vi "周期设置_氨氮.vi"() -> ()   [LabVIEW 2016, in "斯坦道氨氮.lvlib"]
uses:
  <vilib>/Utility/miscctls.llb/LVPointTypeDef.ctl
  <vilib>/Utility/config.llb/NI_LVConfig.lvlib
panel:
  in  "运行周期":T1={"运行模式"=enum."维护模式", "质控频次"=enum."关闭", "空白核查时间"=2, "跨度核查时间"=6, "24H周期设置"=[]} {"跨度核查时间" items=["00H", "01H", "02H", "03H", "04H", "05H", "06H", "07H", "08H", "09H", "10H", "11H", "12H", "13H", "14H", "15H", "16H", "17H", "18H", "19H", "20H", "21H", "22H", "23H", "关闭"]; "空白核查时间" items=["00H", "01H", "02H", "03H", "04H", "05H", "06H", "07H", "08H", "09H", "10H", "11H", "12H", "13H", "14H", "15H", "16H", "17H", "18H", "19H", "20H", "21H", "22H", "23H", "关闭"]}
  # "运行模式："
  # "质控频次："
  # "空白核查时间："
  # "跨度核查时间："
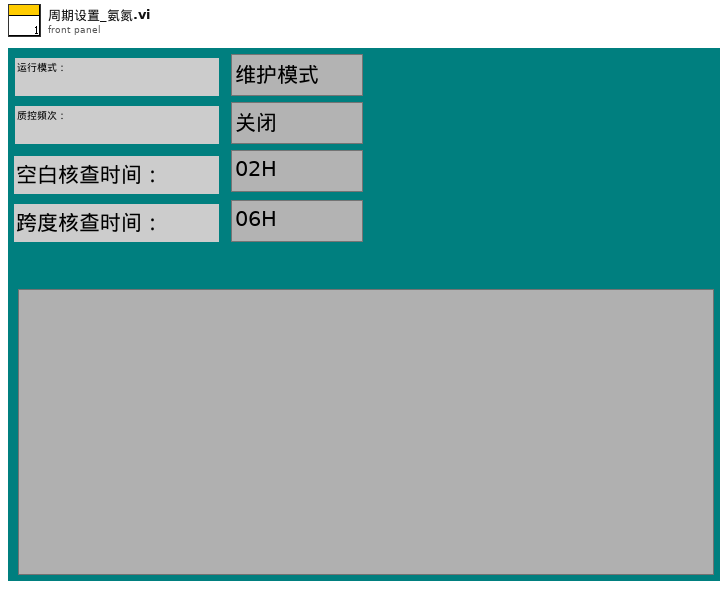
[diagram p1: front panel]
types:
  T1 = cluster{"运行模式":enum16{"维护模式", "常规模式", "应急模式", "质控模式"}, "质控频次":enum16{"关闭", "每天", "星期一", "星期二", "星期三", "星期四", "星期五", "星期六", "星期日"}, "空白核查时间":u16, "跨度核查时间":u16, "24H周期设置":bool[]}
  T2 = typedef "LVPointTypeDef.ctl" = cluster{"Horizontal":i16, "Vertical":i16}
  T3 = cluster{"站号":u16, "量程切换":enum32{"H", "L", "AUTO"}, "控制命令":enum16{"启动测量", "标样核查", "零点核查", "跨度核查", "空白测试", "平行样测试", "加标回收", "空白校准", "标样校准", "初始化（清洗）", "停止测试", "仪器重启", "校时", "模式设置", "测量间隔设置"}, "模式设置":enum16{"待机", "连续模式", "周期模式", "定点模式", "受控模式", "手动模式"}, "测量间隔":u16}
  T4 = enum16{"启动测量", "标样核查", "零点核查", "跨度核查", "空白测试", "平行样测试", "加标回收", "空白校准", "标样校准", "初始化（清洗）", "停止测试", "仪器重启", "校时", "模式设置", "测量间隔设置"}
  T5 = enum16{"关闭", "每天", "星期一", "星期二", "星期三", "星期四", "星期五", "星期六", "星期日"}
  T6 = typedef "LVDateTimeRec.ctl" = cluster{"秒数的小数部分":dbl, "秒":i32, "分":i32, "时":i32, "日":i32, "月":i32, "年":i32, "天数（周）":i32, "天数（年）":i32, "DST":i32}
  T7 = enum32{"Bad", "Idle", "Run top level", "Running"}
  T8 = cluster{"水样测试量程模式":enum16{"H", "L", "AUTO"}, "空白核查量程模式":enum16{"H", "L", "AUTO"}, "跨度核查量程模式":enum16{"H", "L", "AUTO"}}
  T9 = typedef "NI_LVConfig.lvlib/Config Data RefNum.ctl" = refnum<k1>
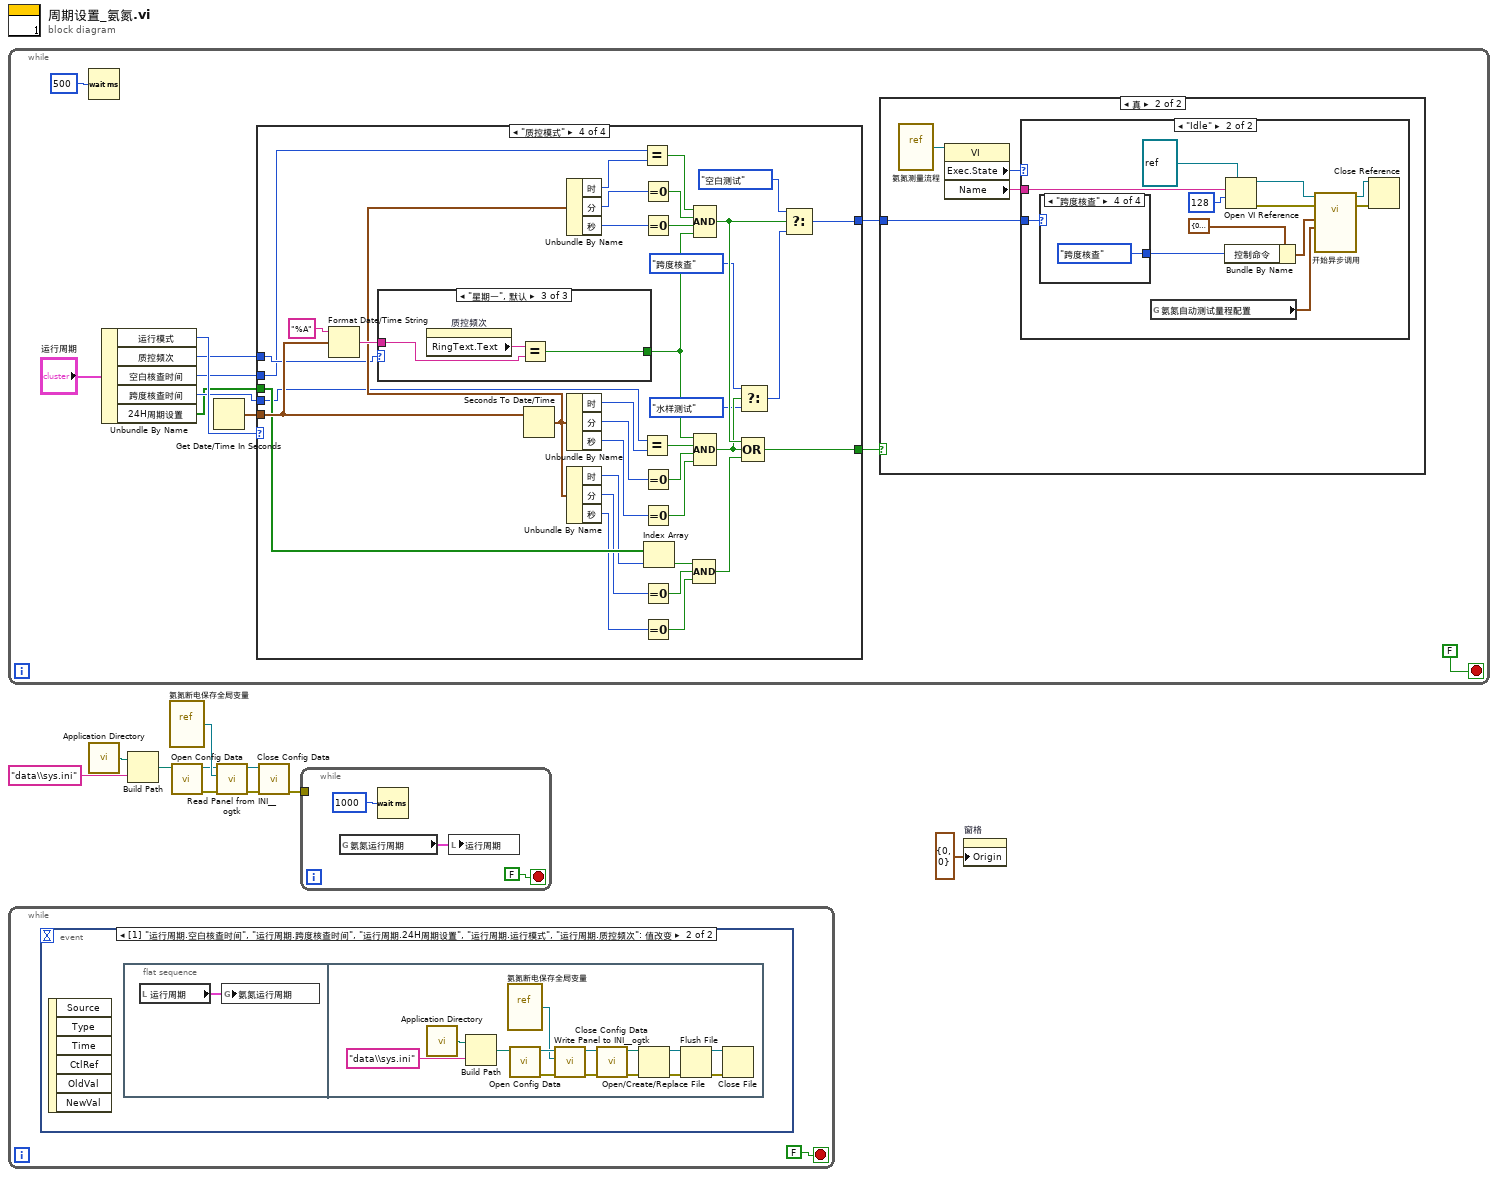
[diagram p0: block diagram]
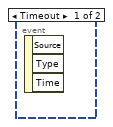
[diagram p2: hidden frame]
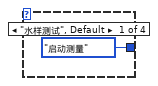
[diagram p5: hidden frame]
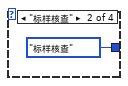
[diagram p6: hidden frame]
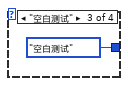
[diagram p7: hidden frame]
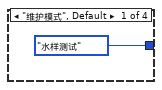
[diagram p8: hidden frame]
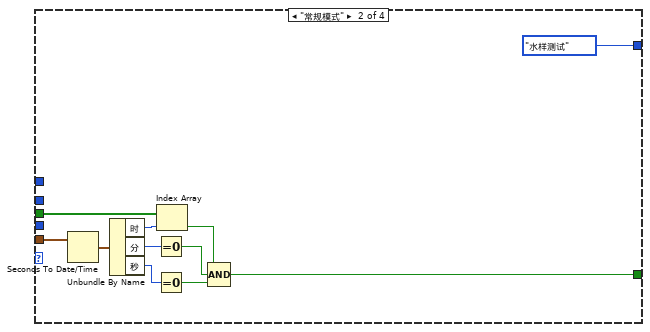
[diagram p9: hidden frame]
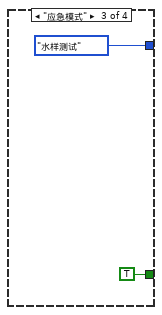
[diagram p10: hidden frame]
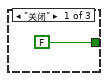
[diagram p11: hidden frame]
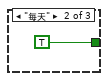
[diagram p12: hidden frame]
diagram:
  n1 = while {
    stop <- FALSE stop-if-true
    n2 = Wait (ms)(milliseconds to wait=u32 500 ("等待时间（毫秒）")) -> ()  [unwired: 1 out]
    n3 = Unbundle By Name("运行周期") -> ("运行模式"=w15:enum16{"维护模式", "常规模式", "应急模式", "质控模式"}, "质控频次"=w14:T5, "空白核查时间"=w13:u16, "跨度核查时间"=w12:u16, "24H周期设置"=w11:bool[])
    n4 = Get Date/Time In Seconds() -> (seconds since 1Jan1904=w21:timestamp)
    n5 = case shown="\"质控模式\"" w15 {
      tunnel: w21 -> [_ w52 _ w91]
      tunnel: w11 -> [_ w49 _ w88]
      tunnel: [_ w43 TRUE w68] -> w18
      tunnel: [enum16{"水样测试", "标样核查", "空白测试", "跨度核查"}."水样测试" ("仪器测试类型") enum16{"水样测试", "标样核查", "空白测试", "跨度核查"}."水样测试" ("仪器测试类型") enum16{"水样测试", "标样核查", "空白测试", "跨度核查"}."水样测试" ("仪器测试类型") w61] -> w17
      tunnel: w14 -> [_ _ _ w58]
      tunnel: w13 -> [_ _ _ w57]
      tunnel: w12 -> [_ _ _ w56]
      frame "维护模式", Default {
      }
      frame "常规模式" {
        n6 = Seconds To Date/Time(time stamp (now)=w52) -> (date time rec=w51:T6)  [unwired: 1 in]
        n7 = Unbundle By Name(w51) -> ("时"=w50:i32, "分"=w48:i32, "秒"=w47:i32)
        n8 = Equal To 0?(x=w48) -> (x = 0?=w45:bool)
        n9 = Equal To 0?(x=w47) -> (x = 0?=w44:bool)
        n10 = Index Array(array=w49, index=w50) -> (element=w46:bool)
        n11 = Compound Arithmetic op=AND ("复合运算")(w46, w45, w44) -> (w43:bool)
      }
      frame "应急模式" {
      }
      frame "质控模式" {
        n12 = Format Date/Time String(time format string (%c)="%A" ("时间格式字符串(%c)"), seconds (now)=w91) -> (date/time string=w89:string)  [unwired: 1 in]
        n13 = case shown="\"星期一\", 默认" w58 {
          tunnel: w89 -> [_ _ w95]
          tunnel: [FALSE TRUE w94] -> w59
          frame "关闭" {
          }
          frame "每天" {
          }
          frame "星期一", Default {
            n14 = property on="质控频次" class="Enum (严格)"() -> ("RingText.Text"=w96:string)  [unwired: 2 in, 2 out]
            n15 = Equal?(x=w96, y=w95) -> (x = y?=w94:bool)
          }
        }
        n16 = Seconds To Date/Time(time stamp (now)=w91) -> (date time rec=w72:T6)  [unwired: 1 in]
        n17 = Unbundle By Name(w72) -> ("时"=w81:i32, "分"=w80:i32, "秒"=w79:i32)
        n18 = Unbundle By Name(w72) -> ("时"=w73:i32, "分"=w74:i32, "秒"=w75:i32)
        n19 = Unbundle By Name(w72) -> ("时"=w87:i32, "分"=w85:i32, "秒"=w83:i32)
        n20 = Equal?(x=w57, y=w81) -> (x = y?=w78:bool)
        n21 = Equal?(x=w56, y=w73) -> (x = y?=w71:bool)
        n22 = Equal To 0?(x=w80) -> (x = 0?=w77:bool)
        n23 = Equal To 0?(x=w79) -> (x = 0?=w76:bool)
        n24 = Equal To 0?(x=w74) -> (x = 0?=w70:bool)
        n25 = Equal To 0?(x=w75) -> (x = 0?=w69:bool)
        n26 = Equal To 0?(x=w85) -> (x = 0?=w84:bool)
        n27 = Equal To 0?(x=w83) -> (x = 0?=w82:bool)
        n28 = Index Array(array=w88, index=w87) -> (element=w86:bool)
        n29 = Compound Arithmetic op=AND ("复合运算")(w86, w84, w82) -> (w60:bool)
        n30 = Compound Arithmetic op=AND ("复合运算")(w78, w77, w76, w59) -> (w67:bool)
        n31 = Compound Arithmetic op=AND ("复合运算")(w59, w71, w70, w69) -> (w65:bool)
        n32 = Select(t=enum16{"水样测试", "标样核查", "空白测试", "跨度核查"}."跨度核查" ("仪器测试类型"), s=w65, f=enum16{"水样测试", "标样核查", "空白测试", "跨度核查"}."水样测试" ("仪器测试类型")) -> (s? t:f=w63:enum16{"水样测试", "标样核查", "空白测试", "跨度核查"})
        n33 = Compound Arithmetic op=OR ("复合运算")(w67, w65, w60) -> (w68:bool)
        n34 = Select(t=enum16{"水样测试", "标样核查", "空白测试", "跨度核查"}."空白测试" ("仪器测试类型"), s=w67, f=w63) -> (s? t:f=w61:enum16{"水样测试", "标样核查", "空白测试", "跨度核查"})
      }
    }
    n35 = case shown="真" w18 {
      tunnel: w17 -> [_ w22]
      frame False {
      }
      frame True {
        n36 = vi-ref "氨氮测量流程.vi"() -> (w23:refnum<vi>)
        n37 = property class="VI"(reference=w23) -> ("Exec.State"=w25:T7, "Name"=w24:string)  [unwired: 1 in, 2 out]
        n38 = case shown="\"Idle\"" w25 {
          tunnel: w24 -> [_ w32]
          tunnel: w22 -> [_ w26]
          frame "Bad", Default {
          }
          frame "Idle" {
            n39 = case shown="\"跨度核查\"" w26 {
              tunnel: [T4."启动测量" ("控制命令") T4."标样核查" ("控制命令") T4."空白测试" ("控制命令") T4."跨度核查" ("控制命令")] -> w28
              frame "水样测试", Default {
              }
              frame "标样核查" {
              }
              frame "空白测试" {
              }
              frame "跨度核查" {
              }
            }
            n40 = global read "氨氮断电保存全局变量.vi" "氨氮自动测试量程配置"() -> (w27:T8)
            n41 = Bundle By Name(cluster=T3 {"站号"=0, "量程切换"=enum."H", "控制命令"=enum."启动测量", "模式设置"=enum."待机", "测量间隔"=0} ("参数"), "控制命令"=w28) -> (w29:T3)
            n42 = Open VI Reference(type specifier VI Refnum (for type only)=refnum<vi> refnum, vi path=w32, options=128 ("选项")) -> (vi reference=w33:refnum<vi>, error out=w34:errorcluster)  [unwired: 3 in]
            n43 = call-by-ref "开始异步调用"(reference=w33, error in=w34, "量程模式"=w27, "参数"=w29) -> (reference out=w35:refnum<vi>, error out=w36:errorcluster)  [unwired: 10 in]
            n44 = Close Reference(reference=w35, error in (no error)=w36) -> ()  [unwired: 1 out]
          }
        }
      }
    }
  }
  n45 = while {
    stop <- FALSE stop-if-true
    n46 = event shown="[1] \"运行周期.空白核查时间\", \"运行周期.跨度核查时间\", \"运行周期.24H周期设置\", \"运行周期.运行模式\", \"运行周期.质控频次\": 值改变" {
      selector: _ -> [_ _]
      dyn-events: _ -> [_ _]
      timeout: _ -> [_ _]
      event Timeout {
        n47 = event-data() -> ()  [unwired: 1 in, 3 out]
      }
      event "运行周期.空白核查时间", "运行周期.跨度核查时间", "运行周期.24H周期设置", "运行周期.运行模式", "运行周期.质控频次": Value Change {
        n48 = event-data() -> ()  [unwired: 1 in, 6 out]
        n49 = flat-sequence {
          frame #0 {
            n50 = local read "运行周期"() -> (w98:T1)
            n51 = global write "氨氮断电保存全局变量.vi" "氨氮运行周期"(w98) -> ()
          }
          frame #1 {
            n52 = call <vilib>:"Application Directory.vi"() -> ("Application Directory"=w112:path)
            n53 = Build Path(base path=w112, name or relative path="data\\sys.ini" ("名称或相对路径")) -> (appended path=w110:path)
            n54 = vi-ref "氨氮断电保存全局变量.vi"() -> (w108:refnum<vi>)
            n55 = call <vilib>:"Open Config Data.vi"("configuration file path"=w110) -> ("error out"=w106:errorcluster, "refnum"=w109:T9)  [unwired: 8 in, 1 out]
            n56 = call <userlib>:"Write Panel to INI__ogtk.vi"("error in (no error)"=w106, "VI ref"=w108, "refnum"=w109) -> ("error out"=w105:errorcluster, "refnum out"=w107:T9)  [unwired: 7 in]
            n57 = call <vilib>:"Close Config Data.vi"("error in (no error)"=w105, "refnum"=w107) -> ("error out"=w100:errorcluster, "file path"=w99:path)  [unwired: 8 in]
            n58 = Open/Create/Replace File(file path (use dialog)=w99, error in=w100) -> (refnum out=w103:refnum<file>, error out=w104:errorcluster)  [unwired: 4 in, 1 out]
            n59 = Flush File(refnum=w103, error in=w104) -> (refnum out=w102:refnum<file>, error out=w101:errorcluster)
            n60 = Close File(refnum=w102, error in=w101) -> ()  [unwired: 2 out]
          }
        }
      }
    }
  }
  n61 = call <vilib>:"Application Directory.vi"() -> ("Application Directory"=w3:path)
  n62 = Build Path(base path=w3, name or relative path="data\\sys.ini" ("名称或相对路径")) -> (appended path=w5:path)
  n63 = vi-ref "氨氮断电保存全局变量.vi"() -> (w7:refnum<vi>)
  n64 = call <vilib>:"Open Config Data.vi"("configuration file path"=w5) -> ("error out"=w9:errorcluster, "refnum"=w6:T9)  [unwired: 8 in, 1 out]
  n65 = call <userlib>:"Read Panel from INI__ogtk.vi"("error in (no error)"=w9, "VI ref"=w7, "refnum"=w6) -> ("error out"=w10:errorcluster, "refnum out"=w8:T9)  [unwired: 7 in]
  n66 = call <vilib>:"Close Config Data.vi"("error in (no error)"=w10, "refnum"=w8) -> ("error out"=w2:errorcluster)  [unwired: 8 in, 1 out]
  n67 = while {
    tunnel: w2 -> [_]
    stop <- FALSE stop-if-true
    n68 = global read "氨氮断电保存全局变量.vi" "氨氮运行周期"() -> (w113:T1)
    n69 = Wait (ms)(milliseconds to wait=u32 1000 ("等待时间（毫秒）")) -> ()  [unwired: 1 out]
    n70 = local write "运行周期"(w113) -> ()
  }
  n71 = property on="窗格" class="Pane"("Origin"=T2 {"Horizontal"=0, "Vertical"=0} ("原点")) -> ()  [unwired: 2 in, 2 out]
